vi "Save Results.vi"(8 "error in (no error)":errorcluster, 10 "Results":refnum<class "Result.lvclass">[](array[class]), 11 "Formatter in":refnum<class "Formatter.lvclass">) -> (0 "error out":errorcluster, 3 "Formatter out":refnum<class "Formatter.lvclass">)   [LabVIEW 2015, in "Formatter.lvclass"]
doc: "This VI will take the array of results, format them and write them to the permanent report."
uses:
  Formatter.lvclass
  Result/Result.lvclass
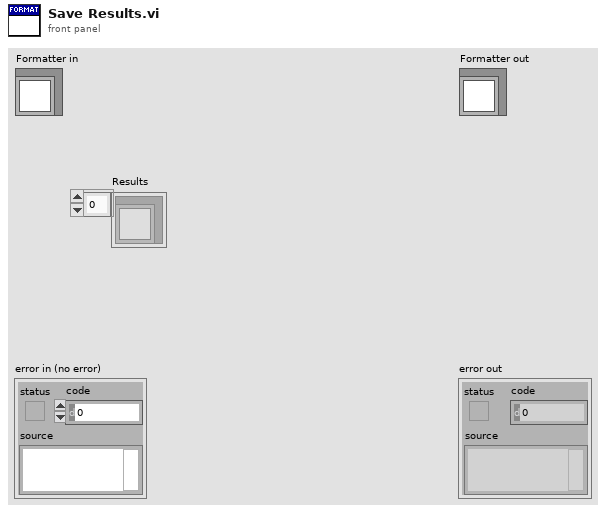
[diagram p1: front panel]
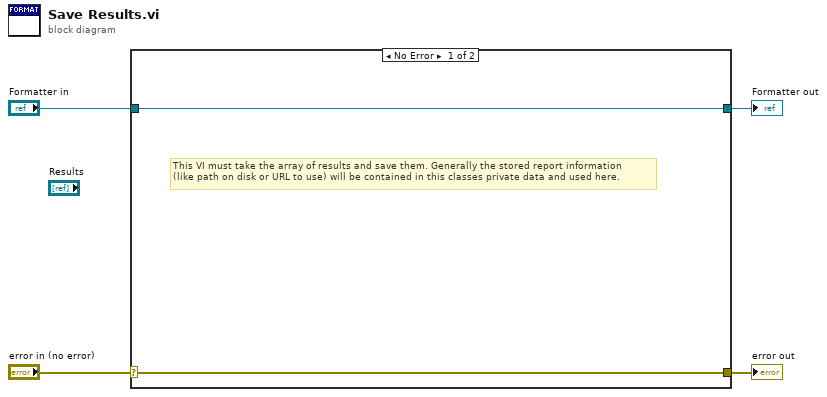
[diagram p0: block diagram]
diagram:
  n1 = case shown="No Error" "error in (no error)" {
    selector: "error in (no error)" -> [w5 w8]
    tunnel: [w5 w8] -> w3
    tunnel: [w6 w7] -> w1
    tunnel: "Formatter in" -> [w6 w7]
    frame No Error {
      # "This VI must take the array of results and save them. Generally the stored report information\n(like path on disk or URL to use) will be contained in this classes private data and used here."
    }
    frame Error {
    }
  }
  "error out" <- w3
  "Formatter out" <- w1
